vi "Initialize.vi"(8 "error in":errorcluster, 10 "parameters":variant, 11 "SwitchACIR Channel in":refnum<class "SwitchACIR Channel.lvclass">) -> (0 "error out":errorcluster, 2 "summary":T2[](array[typedef]), 3 "data value reference":T1)   [LabVIEW 2025, in "SwitchACIR Channel.lvclass"]
doc: "This Vi initializes the data of a node its default state.\nThe object is not created inside of this ViI, beacuase it is created from a File depending on user selection.Copyright 2017 National Instruments Corporation\n\nLicensed under the Apache License, Version 2.0 (the \"License\"); you may not use this file except in compliance with the License. You may obtain a copy of the License at http://www.apache.org/licenses/LICENSE-2.0\nUnless required by applicable law or agreed to in writing, software distributed under the License is distributed on an \"AS IS\" BASIS, WITHOUT WARRANTIES OR CONDITIONS OF ANY KIND, either express or implied. See the License for the specific language governing permissions and limitations under the License."
uses:
  SwitchACIR Channel.lvclass
  C:/Users/Public/Documents/Sandia National Labs/TSS Plugin/CEF.lvlibp/Node/CEF_Node.lvclass
  Users/Public/Documents/Sandia National Labs/TSS Plugin/CEF.lvlibp/Node/Summary.ctl
  Users/Public/Documents/Sandia National Labs/TSS Plugin/CEF.lvlibp/Node/NodeRef.ctl
  Users/Public/Documents/Sandia National Labs/TSS Plugin/CEF.lvlibp/Node/CEF_Node.lvclass
  ACIR Instrument/ACIR Instrument.lvclass
  SwitchACIR Channel.lvclass/SwitchACIR Channel.ctl
  ACIR configuration/ACIR configuration.lvclass
  C:/Users/Public/Documents/Sandia National Labs/TSS Plugin/Abstract Engine.lvlibp/Plugin/Abstract/Instrument configuration/Instrument configuration.lvclass
  SwitchACIR Channel configuration/SwitchACIR Channel configuration.lvclass
  C:/Users/Public/Documents/Sandia National Labs/TSS Plugin/Abstract Engine.lvlibp/Plugin/Abstract/Channel configuration/Channel configuration.lvclass
  Users/Public/Documents/Sandia National Labs/TSS Plugin/CEF.lvlibp/Node/ReadParent.vi
  Users/Public/Documents/Sandia National Labs/TSS Plugin/CEF.lvlibp/Node/ReadChildren.vi
  Users/Public/Documents/Sandia National Labs/TSS Plugin/Abstract Engine.lvlibp/Plugin/Abstract/Instrument configuration/Read Instrument Setting.vi
  Users/Public/Documents/Sandia National Labs/TSS Plugin/Abstract Engine.lvlibp/Plugin/Abstract/Channel configuration/Read Channel Setting.vi
  Users/Public/Documents/Sandia National Labs/TSS Plugin/Abstract Engine.lvlibp/Plugin/Abstract/Channel configuration/Write Channel Setting.vi
  Users/Public/Documents/Sandia National Labs/TSS Plugin/CEF.lvlibp/serializable configuration/CEF_serializable configuration.lvclass
  Users/Public/Documents/Sandia National Labs/TSS Plugin/Abstract Engine.lvlibp/Plugin/Abstract/Abstract Channel/Abstract Channel.lvclass
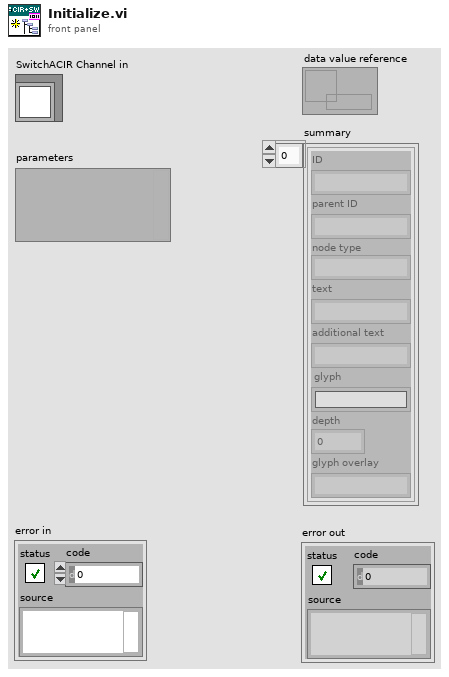
[diagram p1: front panel]
types:
  T1 = typedef "CEF.lvlibp/CEF_Node.lvclass/NodeRef.ctl" = refnum<data-value>
  T2 = typedef "CEF.lvlibp/CEF_Node.lvclass/Summary.ctl" = cluster{"ID":string, "parent ID":string, "node type":string, "text":string, "additional text":string, "glyph":string, "depth":i32, "glyph overlay":string}
  T3 = typedef "Abstract Engine.lvlibp/Instrument configuration.lvclass/Default Instrument.ctl" = cluster{"Type":string, "Address":string, "SW Alias":string, "Description":string, "Enabled":bool}
  T4 = typedef "Abstract Engine.lvlibp/Channel configuration.lvclass/Default Channel.ctl" = cluster{"Address":string, "SW Alias":string, "Enabled":bool, "Type":string, "Description":string}
  T5 = cluster{"ID":string, "parent ID":string, "node type":string, "text":string, "additional text":string, "glyph":string, "depth":i32, "glyph overlay":string}[]
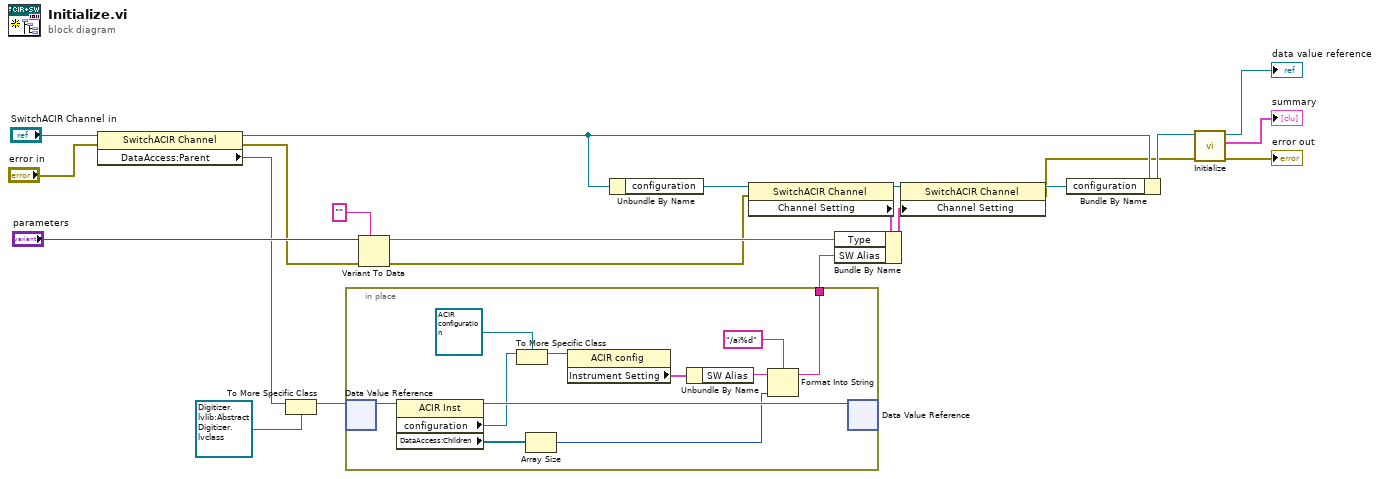
[diagram p0: block diagram]
diagram:
  n1 = property class="SwitchACIR Channel"(reference="SwitchACIR Channel in", error in="error in") -> (reference out=w14:refnum<class "SwitchACIR Channel.lvclass">, error out=w9:errorcluster, "DataAccess:Parent"=w16:refnum<data-value>)
  n2 = To More Specific Class(target class=refnum<data-value> refnum ("data value reference"), reference=w16) -> (specific class reference=w17:refnum<data-value>)  [unwired: 1 in, 1 out]
  n3 = in-place {
    in-place-border: [w31] -> w10
    n4 = in-place-dvr #1(w17) -> (w30:refnum<class "ACIR Instrument.lvclass">)  [unwired: 1 out]
    n5 = property class="ACIR Inst"(reference=w30) -> (reference out=w29:refnum<class "ACIR Instrument.lvclass">, "configuration"=w28:refnum<class "CEF_serializable configuration.lvclass">, "DataAccess:Children"=w27:refnum<data-value>[])  [unwired: 1 in, 1 out]
    n6 = To More Specific Class(target class=refnum<class "ACIR configuration.lvclass"> refnum ("Digitizer.lvlib:Digitizer configuration.lvclass"), reference=w28) -> (specific class reference=w33:refnum<class "ACIR configuration.lvclass">)  [unwired: 1 in, 1 out]
    n7 = Array Size(array=w27) -> (size(s)=w25:i32)
    n8 = property class="ACIR config"(reference=w33) -> ("Instrument Setting"=w24:T3)  [unwired: 1 in, 2 out]
    n9 = Unbundle By Name(w24) -> ("SW Alias"=w32:string)
    n10 = Format Into String(format string="/ai%d", initial string=w32, w25) -> (resulting string=w31:string)  [unwired: 1 in, 1 out]
    n11 = in-place-dvr #1(w29) -> ()  [unwired: 2 out]
  }
  n12 = Variant To Data(error in=w9, type="", Variant="parameters") -> (data=w6:string, error out=w4:errorcluster)
  n13 = Unbundle By Name(w14) -> ("configuration"=w15:refnum<class "SwitchACIR Channel configuration.lvclass">)
  n14 = property class="SwitchACIR Channel"(reference=w15, error in=w4) -> (reference out=w5:refnum<class "SwitchACIR Channel configuration.lvclass">, "Channel Setting"=w3:T4)  [unwired: 1 out]
  n15 = Bundle By Name(cluster=w3, "Type"=w6, "SW Alias"=w10) -> (w2:T4)
  n16 = property class="SwitchACIR Channel"(reference=w5, "Channel Setting"=w2) -> (reference out=w12:refnum<class "SwitchACIR Channel configuration.lvclass">, error out=w8:errorcluster)  [unwired: 1 in]
  n17 = Bundle By Name(cluster=w14, "configuration"=w12) -> (w13:refnum<class "SwitchACIR Channel.lvclass">)
  n18 = call-parent "Initialize.vi"("error in"=w8, "CEF_Serialize node in"=w13) -> ("error out"=→"error out":errorcluster, "summary"=→"summary":T5, "data value reference"=→"data value reference":refnum<data-value>)  [unwired: 7 in]
